vi "Test String to float.vi"() -> ()   [LabVIEW 2017]
panel:
  in  "String":string[](array[string])=["3.14E+5", "3.14E-5", "3.21M", "3.21m", "3.21K", "3.21k", "3.21u", "23.43"]
  out "float":dbl[](array[numeric])=[314000.0, 3.1400000000000004e-05, 3210000.0, 0.00321, 3210.0, 3210.0, 3.2099999999999998e-06, 2343.0] format="%.10f"
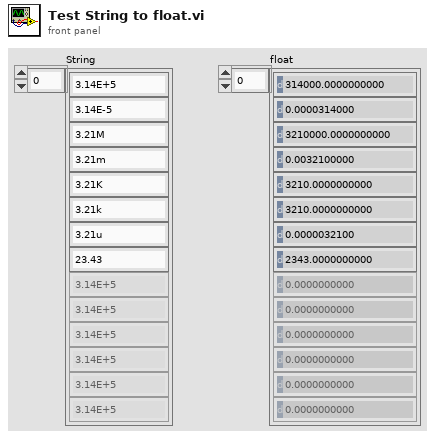
[diagram p1: front panel]
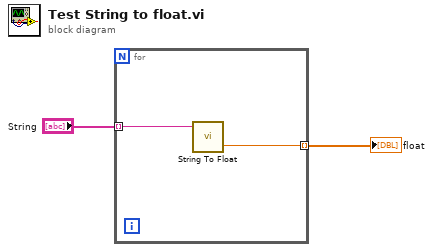
[diagram p0: block diagram]
diagram:
  n1 = for {
    tunnel: "String" -> [w4] mode=indexing
    tunnel: [w3] -> w1 mode=indexing
    n2 = call "String To Float.vi"("String"=w4) -> ("Float"=w3:dbl)  [unwired: 4 in]
  }
  "float" <- w1
